vi "Read Water Level Actor.vi"(11 "Evaporative Cooler":refnum<class "Evaporative Cooler.lvclass">) -> (2 "Water Level":refnum<class "Water Level.lvclass">)   [LabVIEW 2018, in "Evaporative Cooler.lvlib" / "Evaporative Cooler.lvclass"]
doc: "Read the Water Level actor that should be launched by this Evaporative Cooler. Child classes should override this method to return the Water Level that best meets their needs. For example, a simulated evaporative cooler would return a simulated water level."
uses:
  Evaporative Cooler.lvclass
  Water Level/Water Level.lvclass
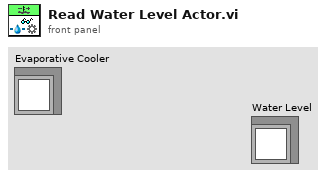
[diagram p1: front panel]
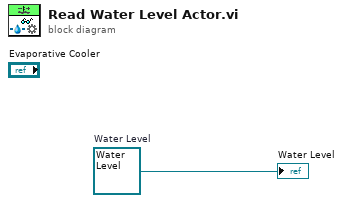
[diagram p0: block diagram]
diagram:
  w1 = refnum<class "Water Level.lvclass"> refnum  # Water Level
  "Water Level" <- w1
